vi "String to Build version.vi"(10 "Build Version (String)":string) -> (3 "Build Version":T1)   [LabVIEW 2021, in "App-Builder Library.lvlib" / "Builder.lvclass"]
uses:
  Builder.lvclass
  <vilib>/AppBuilder/AB_API_Simple/Build Specification Version.ctl
  <vilib>/AppBuilder/AB_API_Simple/NI_App_Builder_API.lvlib
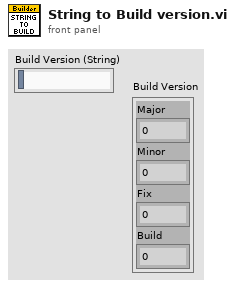
[diagram p1: front panel]
types:
  T1 = typedef "NI_App_Builder_API.lvlib/Build Specification Version.ctl" = cluster{"Major":u16, "Minor":u16, "Fix":u16, "Build":u16}
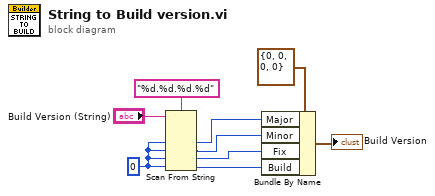
[diagram p0: block diagram]
diagram:
  w2 = u16 0 ("Build")
  n1 = Scan From String(format string="%d.%d.%d.%d", input string="Build Version (String)", default 1=w2, default 2=w2, default 3=w2, default 4=w2) -> (output 1=w6:u16, output 2=w4:u16, output 3=w3:u16, output 4=w1:u16)  [unwired: 2 in, 3 out]
  n2 = Bundle By Name(cluster=T1 {"Major"=0, "Minor"=0, "Fix"=0, "Build"=0} ("Build Version"), "Major"=w6, "Minor"=w4, "Fix"=w3, "Build"=w1) -> (→"Build Version":T1)
